vi "Get Robot Pose.vi"(11 "Detection Robot":T1 {"height" format="%+4.3f"; "pixel_y" format="%+4.3f"; "pixel_x" format="%+4.3f"; "orientation" format="%+4.3f"; "y" format="%+4.3f"; "confidence" format="%4.3f"; "x" format="%+4.3f"}) -> (3 "Pose":sgl[](array[numeric]))   [LabVIEW 2016]
uses:
  SSL Detection Robot.ctl
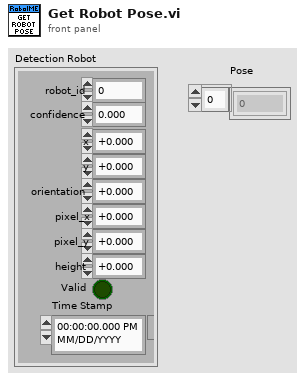
[diagram p1: front panel]
types:
  T1 = typedef "SSL Detection Robot.ctl" = cluster{"x":sgl, "robot_id":u32, "confidence":sgl, "y":sgl, "orientation":sgl, "pixel_x":sgl, "pixel_y":sgl, "height":sgl, "Valid":bool, "Time Stamp":timestamp}
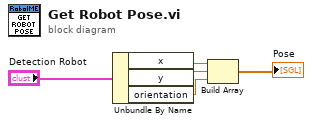
[diagram p0: block diagram]
diagram:
  n1 = Unbundle By Name("Detection Robot") -> ("x"=w2:sgl, "y"=w3:sgl, "orientation"=w4:sgl)
  n2 = Build Array(w2, w3, w4) -> (→"Pose":sgl[])
